vi "Do Attacks.vi"(6 "Teams in":refnum<class "Team.lvclass">[](array[class]), 9 "New Map in":refnum<class "Map.lvclass">) -> (1 "New Map out":refnum<class "Map.lvclass">, 4 "Teams out":refnum<class "Team.lvclass">[](array[class]))   [LabVIEW 2020, in "SquareBattle.lvlib" / "Map.lvclass"]
uses:
  Map.lvclass
  Team/Team.lvclass
  Map.lvclass/Map.ctl
  Square/Square.lvclass
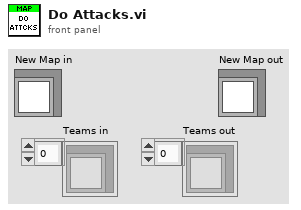
[diagram p1: front panel]
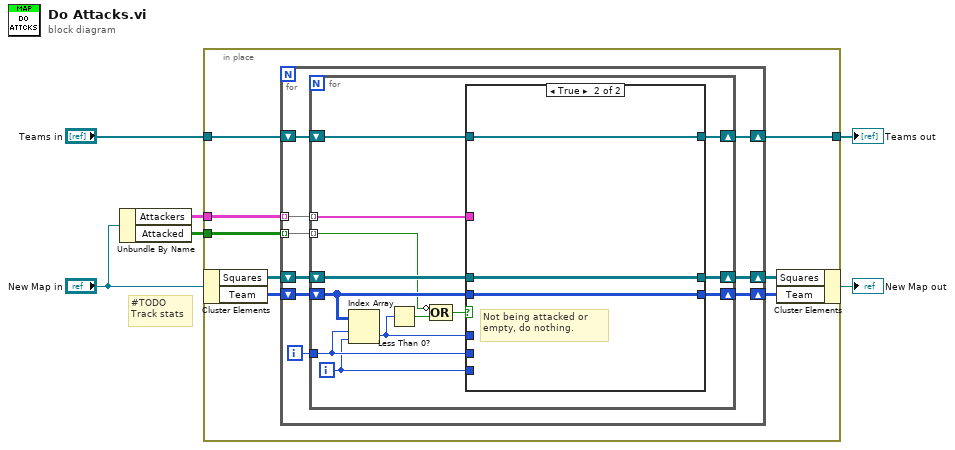
[diagram p0: block diagram]
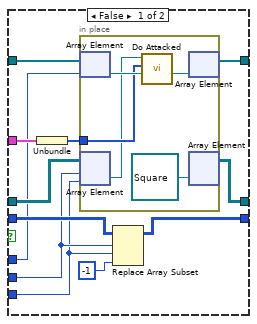
[diagram p2: hidden frame]
diagram:
  # "#TODO\nTrack stats"
  n1 = Unbundle By Name("New Map in") -> ("Attackers"=w1:cluster{"Array":i32[]}[][], "Attacked"=w5:bool[][])
  n2 = in-place {
    in-place-border: w5 -> [w12]
    in-place-border: "Teams in" -> [w11]
    in-place-border: [w10] -> w3
    in-place-border: w1 -> [w7]
    n3 = in-place-cluster #1("New Map in") -> ("Squares"=w14:refnum<class "Square.lvclass">[][], "Team"=w13:i32[][])
    n4 = for {
      shift-right: [w17] -> w8
      shift-left: w13 -> [w22]
      shift-right: [w18] -> w9
      shift-left: w14 -> [w23]
      tunnel: w12 -> [w21] mode=indexing
      shift-right: [w16] -> w10
      shift-left: w11 -> [w20]
      tunnel: w7 -> [w15] mode=indexing
      i -> [w19]
      n5 = for {
        shift-right: [w29] -> w18
        shift-left: w23 -> [w35]
        shift-right: [w30] -> w17
        shift-left: w22 -> [w36]
        tunnel: w21 -> [w32] mode=indexing
        shift-right: [w27] -> w16
        shift-left: w20 -> [w28]
        tunnel: w19 -> [w26]
        tunnel: w15 -> [w24] mode=indexing
        i -> [w25]
        n6 = Index Array(array=w36, index (row)=w26, index (col)=w25) -> (element=w34:i32)
        n7 = Less Than 0?(x=w34) -> (x < 0?=w33:bool)
        n8 = Compound Arithmetic op=OR(invert w32, w33) -> (w31:bool)
        n9 = case shown="True" w31 {
          tunnel: w36 -> [w42 w56]
          tunnel: w35 -> [w45 w55]
          tunnel: w34 -> [w37 _]
          tunnel: [w41 w56] -> w30
          tunnel: [w44 w55] -> w29
          tunnel: w28 -> [w47 w54]
          tunnel: [w43 w54] -> w27
          tunnel: w26 -> [w40 _]
          tunnel: w25 -> [w39 _]
          tunnel: w24 -> [w48 _]
          frame False {
            n10 = Unbundle(w48) -> ("Array"=w46:i32[])
            n11 = in-place {
              in-place-border: w46 -> [w51]
              n12 = in-place-array #2(w47, w37) -> (w52:refnum<class "Team.lvclass">)
              n13 = in-place-array #3(w45, w40, w39) -> (w50:refnum<class "Square.lvclass">)
              n14 = call "Do Attacked.vi"("Team In"=w52, "Attackers"=w51, "Square"=w50) -> ("Team out"=w49:refnum<class "Team.lvclass">)  [unwired: 8 in]
              n15 = in-place-array #2(w49) -> (w43:refnum<class "Team.lvclass">[])  [unwired: 1 out]
              n16 = in-place-array #3(refnum<class "Square.lvclass"> refnum ("element")) -> (w44:refnum<class "Square.lvclass">[][])  [unwired: 2 out]
            }
            n17 = Replace Array Subset(array=w42, new element=-1 ("new element/subarray"), index (row)=w40, index (col)=w39) -> (w41:i32[][])
          }
          frame True {
            # "Not being attacked or empty, do nothing."
          }
        }
      }
    }
    n18 = in-place-cluster #1("Squares"=w9, "Team"=w8) -> (→"New Map out":refnum<class "Map.lvclass">)
  }
  "Teams out" <- w3
